vi "get_featurestudio_features.vi"(0 "Device In":T2, 11 "error in":errorcluster) -> (4 "Device Out":T2, 6 "Comm":T1, 15 "error out":errorcluster)   [LabVIEW 2019]
uses:
  <userlib>/IoT Devices/_subVIs/HTTPComm.ctl
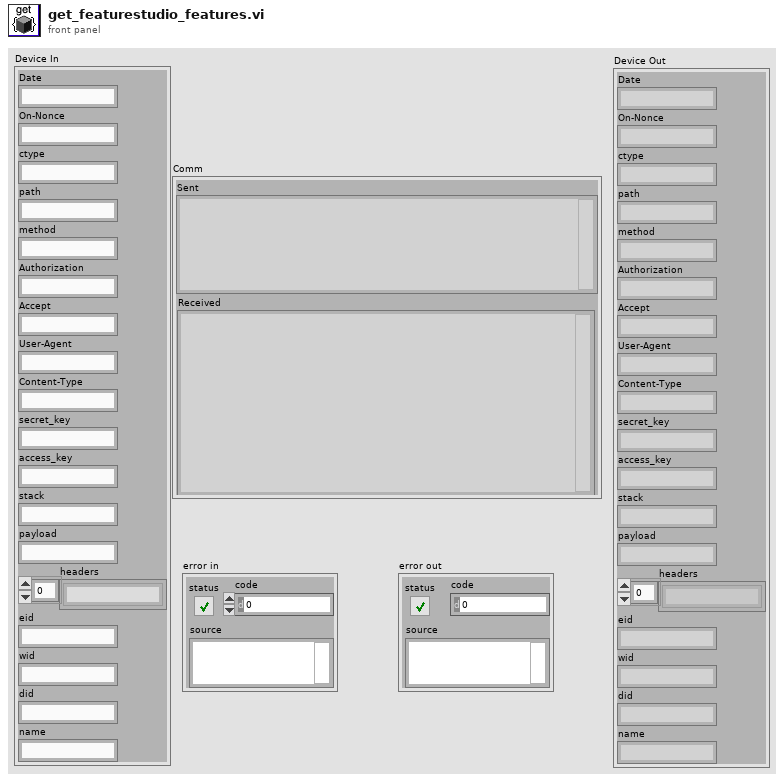
[diagram p1: front panel]
types:
  T1 = typedef "HTTPComm.ctl" = cluster{"url":string, "sent headers":string, "sent body":string, "headers":string, "body":string, "Sent":string, "Received":string}
  T2 = cluster{"Date":string, "On-Nonce":string, "ctype":string, "path":string, "method":string, "Authorization":string, "Accept":string, "User-Agent":string, "Content-Type":string, "secret_key":string, "access_key":string, "stack":string, "payload":string, "headers":string[], "eid":string, "wid":string, "did":string, "name":string}
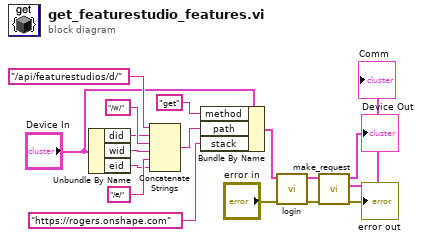
[diagram p0: block diagram]
diagram:
  n1 = Unbundle By Name("Device In") -> ("did"=w4:string, "wid"=w3:string, "eid"=w2:string)
  n2 = Concatenate Strings("/api/featurestudios/d/" ("payload"), w4, "/w/" ("string"), w3, "/e/" ("string"), w2) -> (w13:string)
  n3 = Bundle By Name(cluster="Device In", "method"="get" ("Method"), "path"=w13, "stack"="https://rogers.onshape.com" ("stacks")) -> (w9:T2)
  n4 = call "login.vi"("error in"="error in", "Device In"=w9) -> ("error out"=w7:errorcluster, "Device Out"=w11:T2)  [unwired: 8 in]
  n5 = call "make_request.vi"("Error in"=w7, "Device In"=w11) -> ("error out"=→"error out":errorcluster, "Comm"=→"Comm":T1, "Device Out"=→"Device Out":T2)  [unwired: 7 in]
